vi "Write m1CoverMove.vi"(8 "error in (no error)":errorcluster, 10 "coverMoveTypes":T1, 11 "M1Cover in":refnum<class "M1Cover.lvclass">) -> (0 "error out":errorcluster, 3 "M1Cover out":refnum<class "M1Cover.lvclass">)   [LabVIEW 2014, in "TCSDataDefinitions.lvlib" / "TCSCommand.lvlib" / "M1Cover.lvclass"]
uses:
  M1Cover.lvclass
  Enumerations/M1CoverMoveTypes.ctl
  M1Cover.lvclass/M1Cover.ctl
  TCSCommand.lvlib
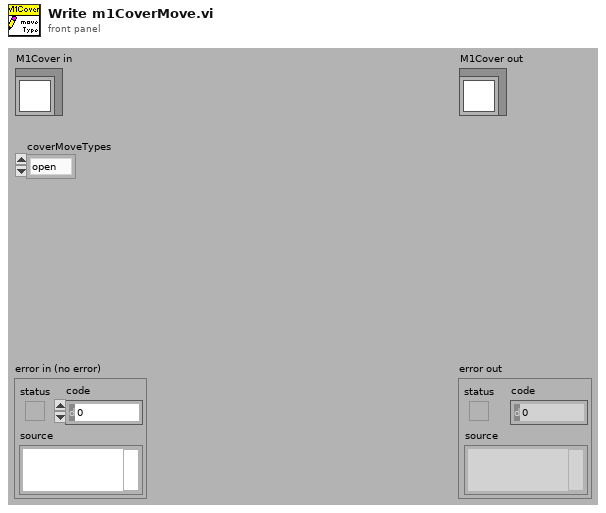
[diagram p1: front panel]
types:
  T1 = typedef "TCSDataDefinitions.lvlib/TCSCommand.lvlib/M1CoverMoveTypes.ctl" = enum16{"open", "close", "stop"}
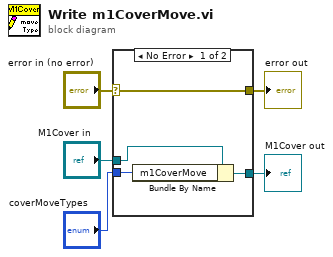
[diagram p0: block diagram]
diagram:
  n1 = case shown="No Error" "error in (no error)" {
    selector: "error in (no error)" -> [w9 w10]
    tunnel: [w9 w10] -> w4
    tunnel: [w7 w11] -> w2
    tunnel: "M1Cover in" -> [w8 w11]
    tunnel: "coverMoveTypes" -> [w6 _]
    frame No Error {
      n2 = Bundle By Name(cluster=w8, "m1CoverMove"=w6) -> (w7:refnum<class "M1Cover.lvclass">)
    }
    frame Error {
    }
  }
  "error out" <- w4
  "M1Cover out" <- w2
